vi "READ_SENSOR.vi"() -> ()   [LabVIEW 2018]
uses:
  <vilib>/Instr/_visa.llb/VISA Configure Serial Port (Instr).vi
panel:
  out "RGB":u8[](array[numeric])
  out "error out":errorcluster
  out "t":u8[](array[numeric]) format="%x"
  out "DATA":u8[](array[numeric]) format="%x"
  out "return count":u32
  in  "stop":bool
  out "read buffer":string
  # "00 0\n10 1\n01 1\n11 0"
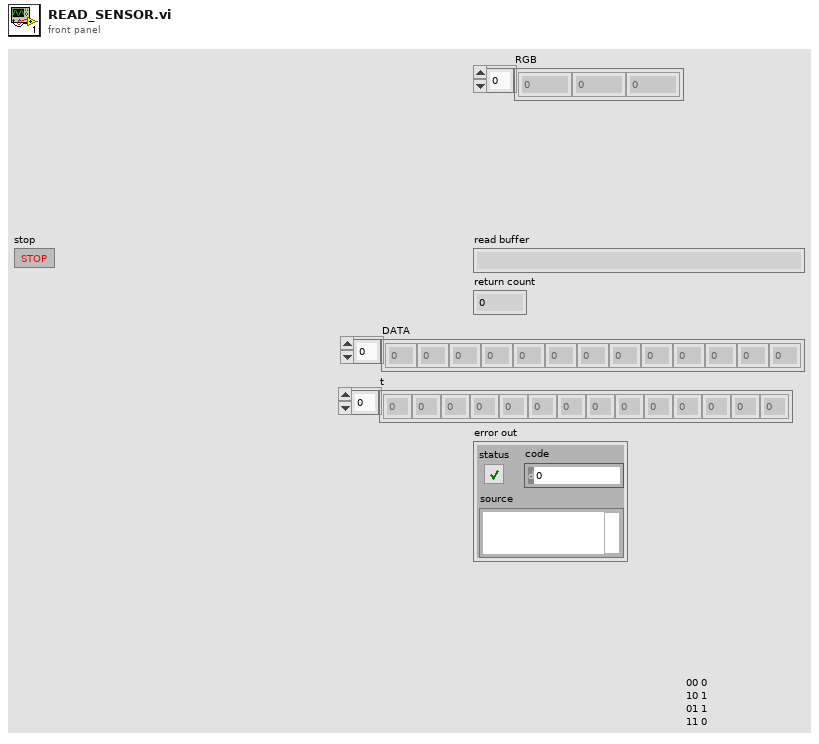
[diagram p1: front panel]
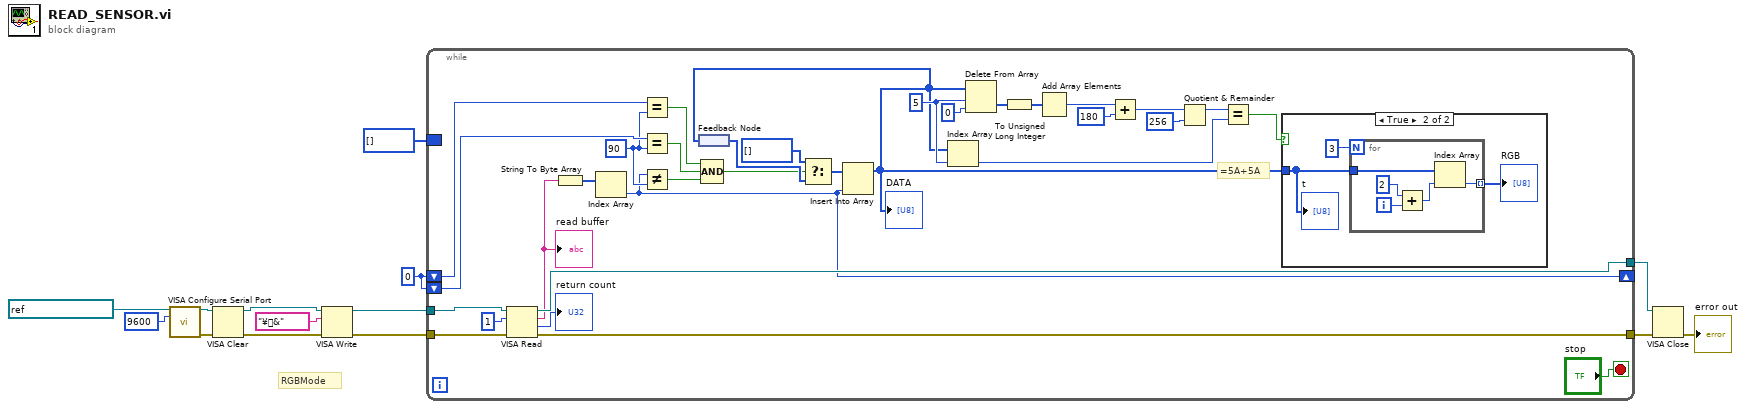
[diagram p0: block diagram]
diagram:
  w10 = u8 0
  # "RGBMode"
  n1 = call-poly "VISA Configure Serial Port"("VISA resource name"=refnum<visa-resource-name> "ASRL1::INSTR", "baud rate (9600)"=u32 9600) -> ("VISA resource name out"=w5:refnum<visa-resource-name>, "error out"=w1:errorcluster)  [unwired: 12 in]
  n2 = VISA Clear(VISA resource name=w5, error in (no error)=w1) -> (VISA resource name out=w4:refnum<visa-resource-name>, error out=w3:errorcluster)
  n3 = VISA Write(VISA resource name=w4, write buffer="¥&", error in (no error)=w3) -> (VISA resource name out=w8:refnum<visa-resource-name>, error out=w7:errorcluster)  [unwired: 1 out]
  n4 = while {
    tunnel: w8 -> [w46]
    tunnel: [w44] -> w12
    border: u8[] [] -> [_]
    shift-right: [w29] -> _
    shift-left: w10 -> [w39]
    shift-left: w10 -> [w38]
    tunnel: w7 -> [w16]
    tunnel: [w15] -> w6
    stop <- "stop" stop-if-true
    w28 = 5 ("index")
    w37 = u8 90 ("y")
    # "=5A+5A"
    n5 = VISA Read(VISA resource name=w46, byte count=u32 1, error in (no error)=w16) -> (VISA resource name out=w44:refnum<visa-resource-name>, read buffer=w41:string, return count=→"return count":u32, error out=w15:errorcluster)
    "read buffer" <- w41
    n6 = String To Byte Array(string=w41) -> (unsigned byte array=w40:u8[])
    n7 = Index Array(array=w40) -> (element=w29:u8)  [unwired: 1 in]
    n8 = Equal?(x=w39, y=w37) -> (x = y?=w36:bool)
    n9 = Equal?(x=w38, y=w37) -> (x = y?=w35:bool)
    n10 = Not Equal?(x=w29, y=w37) -> (x != y?=w34:bool)
    n11 = feedback #1() -> (w33:u8[])
    n12 = Compound Arithmetic op=AND(w36, w35, w34) -> (w30:bool)
    n13 = Select(t=u8[] [], s=w30, f=w33) -> (s? t:f=w31:u8[])
    n14 = Insert Into Array(array=w31, new element=w29) -> (w20:u8[])  [unwired: 1 in]
    "DATA" <- w20
    n15 = feedback-in #1(w20) -> ()
    n16 = Index Array(array=w20, index=w28) -> (element=w22:u8)
    n17 = Delete From Array(array=w20, length=w28, index=0) -> (deleted portion=w26:u8[])  [unwired: 1 out]
    n18 = To Unsigned Long Integer(number=w26) -> (unsigned 32bit integer=w25:u32[])
    n19 = Add Array Elements(numeric array=w25) -> (sum=w19:u32)
    n20 = Add(x=w19, y=u32 180) -> (x+y=w17:u32)
    n21 = Quotient & Remainder(x=w17, y=u32 256) -> (x-y*floor(x/y)=w23:u32)  [unwired: 1 out]
    n22 = Equal?(x=w23, y=w22) -> (x = y?=w21:bool)
    n23 = case shown="True" w21 {
      tunnel: w20 -> [_ w48]
      frame False {
      }
      frame True {
        n24 = for {
          N: 3 -> [_]
          tunnel: w48 -> [w54]
          tunnel: [w50] -> w47 mode=indexing
          i -> [w52]
          n25 = Add(x=2 ("y"), y=w52) -> (x+y=w51:i32)
          n26 = Index Array(array=w54, index=w51) -> (element=w50:u8)
        }
        "RGB" <- w47
        "t" <- w48
      }
    }
  }
  n27 = VISA Close(VISA resource name=w12, error in (no error)=w6) -> (error out=→"error out":errorcluster)
